vi "LoadFromINI.vi"(8 "error in (no error)":errorcluster, 10 "path":path, 11 "reference in":refnum<class "sim_MmW.lvclass">) -> (0 "error out":errorcluster, 3 "reference out":refnum<class "sim_MmW.lvclass">)   [LabVIEW 2019, in "sim_MmW.lvclass"]
doc: "Loads insturment data from ini file"
uses:
  sim_MmW.lvclass
  <vilib>/Utility/error.llb/Error Cluster From Error Code.vi
  <vilib>/ErrorRing/Error Ring.xnode
  <vilib>/Utility/config.llb/NI_LVConfig.lvlib
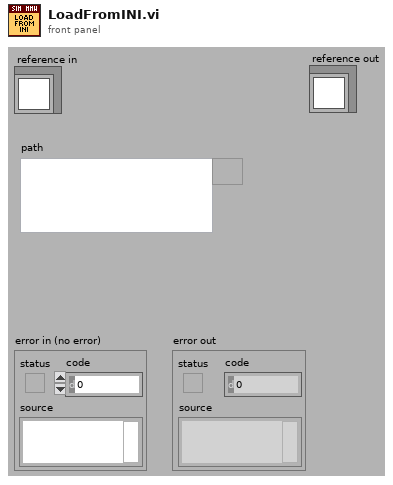
[diagram p1: front panel]
types:
  T1 = typedef "sim_MmW.lvclass/ObjectAttributesRef.ctl" = refnum<data-value>
  T2 = typedef "NI_LVConfig.lvlib/Config Data RefNum.ctl" = refnum<k1>
  T3 = typedef "sim_MmW.lvclass/ObjectAttributes.ctl" = cluster{"RF config":T4, "RX samples":i32, "Downloaded Bursts":map{string, refnum<class "mmWave data.lvclass">}, "TX Fs":dbl, "RX Fs":dbl, "burst sequence":string[], "Burst mode":T5}
  T4 = typedef "mmWave HW Control.lvlib/HW TXRX RF config cluster.ctl" = cluster{"TX.Frequency":dbl, "TX.Gain":dbl, "TX.mmWave adapter":string, "RX.Frequency":dbl, "RX.Gain":dbl, "RX.mmWave adapter":string}
  T5 = typedef "mmWave instrument.lvclass/BurstMode.ctl" = enum16{"burst", "continuous"}
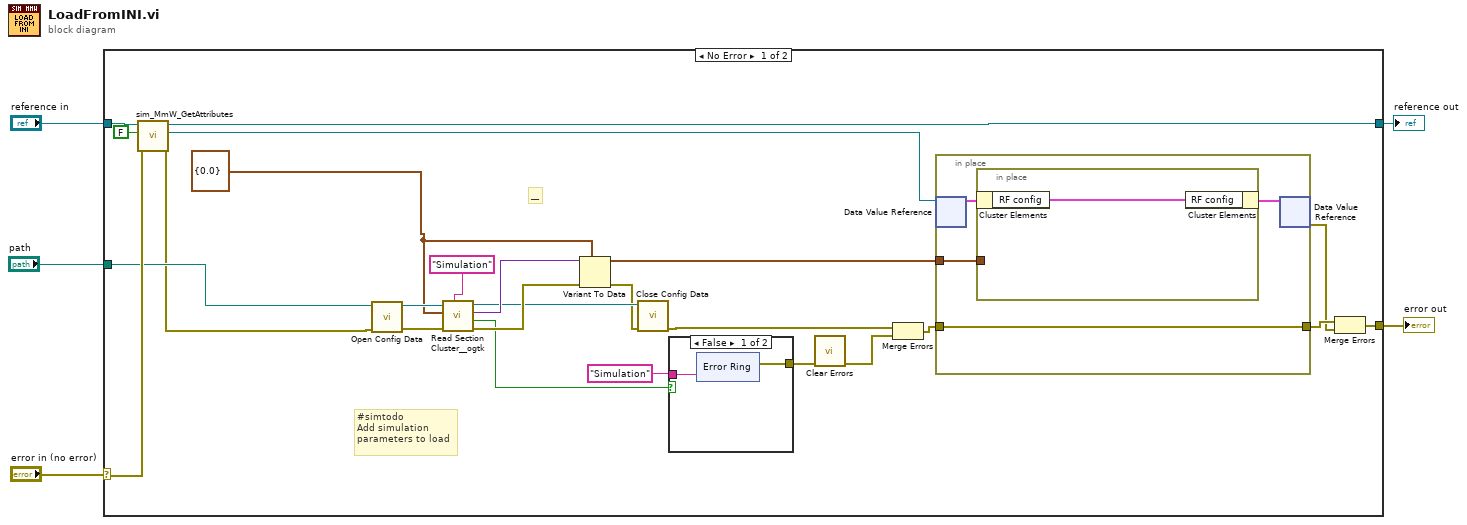
[diagram p0: block diagram]
diagram:
  n1 = case shown="No Error" "error in (no error)" {
    selector: "error in (no error)" -> [w27 w46]
    tunnel: [w30 w46] -> w4
    tunnel: [w28 w45] -> w2
    tunnel: "reference in" -> [w29 w45]
    tunnel: "path" -> [w17 _]
    frame No Error {
      w7 = cluster{"range":dbl} {"range"=0.0}
      # "#simtodo\nAdd simulation\nparameters to load"
      # "__"
      n2 = call "sim_MmW_GetAttributes.vi"("error in (no error)"=w27, "return data? (T)"=FALSE, "reference in"=w29) -> ("error out"=w8:errorcluster, "attributes ref"=w24:T1, "reference out"=w28:refnum<class "sim_MmW.lvclass">)  [unwired: 5 in, 1 out]
      n3 = call <vilib>:"Open Config Data.vi"("error in (no error)"=w8, "configuration file path"=w17) -> ("error out"=w21:errorcluster, "refnum"=w22:T2)  [unwired: 7 in, 1 out]
      n4 = call <userlib>:"Read Section Cluster__ogtk.vi"("section (optional)"="Simulation", "error in (no error)"=w21, "Section Formatted Cluster Type"=w7, "refnum"=w22) -> ("error out"=w19:errorcluster, "all found?"=w16:bool, "Section Formatted Cluster"=w20:variant, "dup refnum"=w12:T2)  [unwired: 3 in, 1 out]
      n5 = Variant To Data(error in=w19, type=w7, Variant=w20) -> (data=w13:cluster{"range":dbl}, error out=w11:errorcluster)
      n6 = call <vilib>:"Close Config Data.vi"("error in (no error)"=w11, "refnum"=w12) -> ("error out"=w10:errorcluster)  [unwired: 8 in, 1 out]
      n7 = case shown="False" w16 {
        tunnel: "Simulation" ("section (optional)") -> [w37 _]
        tunnel: [w36 _] -> w14
        frame False {
          n8 = xnode "Error Ring"("parameter 0"=w37) -> ("error out"=w36:errorcluster)
        }
        frame True {
        }
      }
      n9 = call <vilib>:"Clear Errors.vi"("error in (no error)"=w14) -> ("error out"=w6:errorcluster)  [unwired: 5 in, 1 out]
      n10 = Merge Errors(w10, w6) -> (w9:errorcluster)
      n11 = in-place {
        in-place-border: w9 -> [w32]
        in-place-border: [w32] -> w26
        in-place-border: w13 -> [w31]
        n12 = in-place-dvr #1(w24) -> (w33:T3)  [unwired: 1 out]
        n13 = in-place {
          in-place-border: w31 -> [_]
          n14 = in-place-cluster #2(w33) -> ("RF config"=w35:T4)
          n15 = in-place-cluster #2("RF config"=w35) -> (w34:T3)
        }
        n16 = in-place-dvr #1(w34) -> (w25:errorcluster)  [unwired: 1 out]
      }
      n17 = Merge Errors(w26, w25) -> (w30:errorcluster)
    }
    frame Error {
    }
  }
  "error out" <- w4
  "reference out" <- w2
